vi "Configure Precision Analysis.vi"(8 "error in (no error)":errorcluster, 9 "Analysis Record Length (100000)":i32=100000, 10 "Enable Precision Analysis (T: Enable)":bool=TRUE, 11 "VISA resource name":refnum<visa-resource-name>) -> (0 "error out":errorcluster, 3 "VISA resource name out":refnum<visa-resource-name>)   [LabVIEW 2017, in "Agilent 2000 3000 X-Series.lvlib"]
doc: "Enables and configures the oscilloscope's precision analysis feature.\n\n<b>Note:</b>\nThis VI is specific to the 6000-X Series oscilloscopes. These features are not available on other models."
uses:
  Agilent 2000 3000 X-Series.lvlib
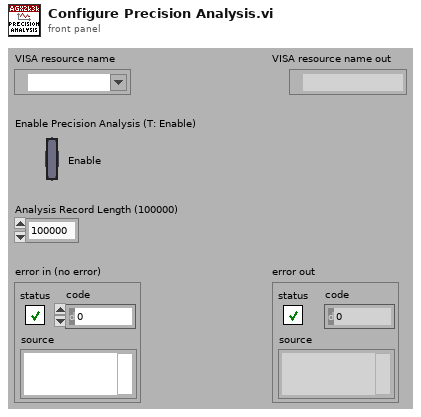
[diagram p1: front panel]
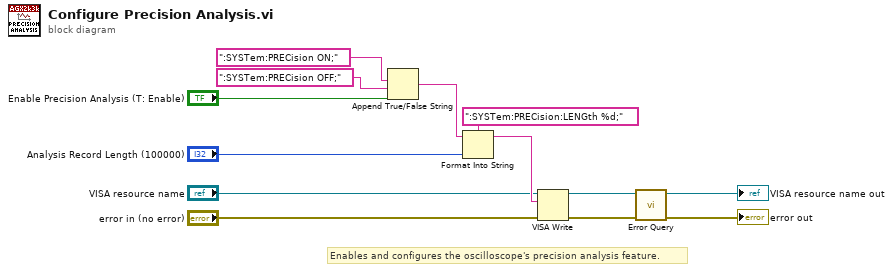
[diagram p0: block diagram]
diagram:
  # "Enables and configures the oscilloscope's precision analysis feature."
  n1 = Append True/False String(1:"Enable Precision Analysis (T: Enable)", 2:":SYSTem:PRECision OFF;", 3:":SYSTem:PRECision ON;") -> (0:w10:string)  [unwired: 1 in]
  n2 = Format Into String(format string=":SYSTem:PRECision:LENGth %d;", initial string=w10, "Analysis Record Length (100000)") -> (resulting string=w7:string)  [unwired: 1 in, 1 out]
  n3 = VISA Write(VISA resource name="VISA resource name", write buffer=w7, error in (no error)="error in (no error)") -> (VISA resource name out=w4:refnum<visa-resource-name>, error out=w3:errorcluster)  [unwired: 1 out]
  n4 = call "Error Query.vi"("error in (no error)"=w3, "VISA resource name"=w4) -> ("error out"=→"error out":errorcluster, "VISA resource name out"=→"VISA resource name out":refnum<visa-resource-name>)  [unwired: 6 in, 2 out]
